vi "Traverse Get Positions.vi"(8 "error in":errorcluster, 10 "VISA resource name":refnum<visa-resource-name>, 11 "Water Tunnel Results in":refnum<class "Water Tunnel Results.lvclass">) -> (0 "error out":errorcluster, 1 "Trav Probe":cluster{"Px":dbl, "Py":dbl, "Pz":dbl}, 2 "Trav Wing":cluster{"Wx":dbl, "Wy":dbl, "Wz":dbl}, 3 "Water Tunnel Results out":refnum<class "Water Tunnel Results.lvclass">)   [LabVIEW 2019, in "Results.lvlib" / "Water Tunnel Results.lvclass"]
uses:
  Water Tunnel Results.lvclass
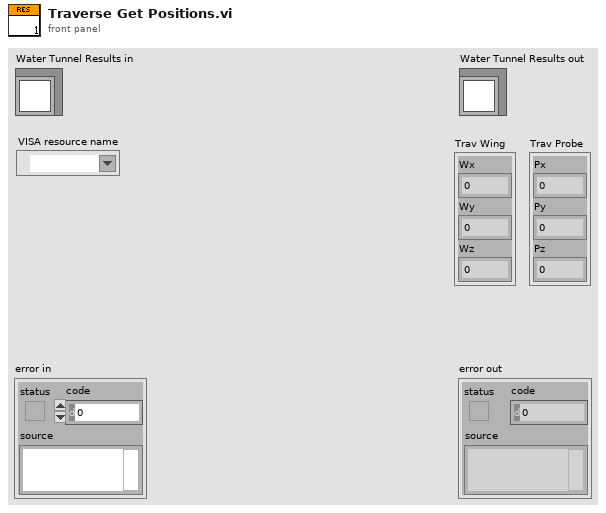
[diagram p1: front panel]
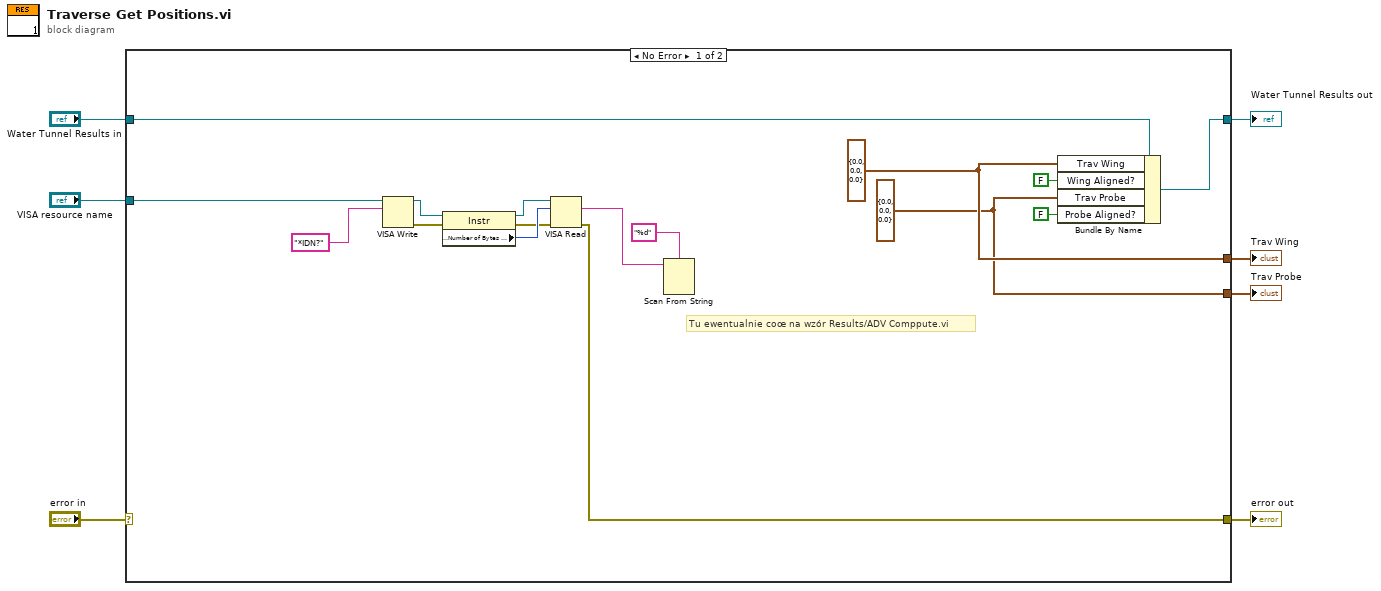
[diagram p0: block diagram]
diagram:
  n1 = case shown="No Error" "error in" {
    selector: "error in" -> [_ w25]
    tunnel: [w8 w25] -> w6
    tunnel: [w19 w24] -> w4
    tunnel: "Water Tunnel Results in" -> [w20 w24]
    tunnel: "VISA resource name" -> [w16 _]
    tunnel: [w10 _] -> w2
    tunnel: [w9 _] -> w1
    frame No Error {
      w9 = cluster{"Px":dbl, "Py":dbl, "Pz":dbl} {"Px"=0.0, "Py"=0.0, "Pz"=0.0} ("Trav Probe")
      w10 = cluster{"Wx":dbl, "Wy":dbl, "Wz":dbl} {"Wx"=0.0, "Wy"=0.0, "Wz"=0.0} ("Trav Wing")
      # "Tu ewentualnie coœ na wzór Results/ADV Comppute.vi"
      n2 = VISA Write(VISA resource name=w16, write buffer="*IDN?") -> (VISA resource name out=w17:refnum<visa-resource-name>, error out=w18:errorcluster)  [unwired: 1 in, 1 out]
      n3 = property class="Instr"(reference=w17, error in=w18) -> (reference out=w23:refnum<visa-resource-name>, error out=w21:errorcluster, "Serial Settings:Number of Bytes at Serial Port"=w22:u32)
      n4 = VISA Read(VISA resource name=w23, byte count=w22, error in (no error)=w21) -> (read buffer=w14:string, error out=w8:errorcluster)  [unwired: 2 out]
      n5 = Scan From String(format string="%d", input string=w14) -> ()  [unwired: 4 in, 3 out]
      n6 = Bundle By Name(cluster=w20, "Trav Wing"=w10, "Wing Aligned?"=FALSE, "Trav Probe"=w9, "Probe Aligned?"=FALSE) -> (w19:refnum<class "Water Tunnel Results.lvclass">)
    }
    frame Error {
    }
  }
  "error out" <- w6
  "Water Tunnel Results out" <- w4
  "Trav Wing" <- w2
  "Trav Probe" <- w1
